vi "Licence Key Generator.vi"() -> ()   [LabVIEW 2013]
panel:
  in  "generator version":string="Version: A (proto) "
  in  "targed directory":path=path "C:/Licences"
  in  "CPU ID":string="AA13E3D1E2B87CC1" caption="Processor ID"
  in  "HDD serial":string="4J810037XGJ2AE" caption="Disk Drive Serial Number"
  in  "application name":string(combo)="Dave.exe" caption="Application name"
  in  "user name":string="Stanley Kubrick" caption="User name"
  in  "machine name":string="Hal 9000" caption="Machine name"
  in  "UUID":string="DB0CF264-5C22-497A-AB4E-F286BC2ADD07" caption="System UUID"
  in  "features":T1={"Feature 1"=TRUE, "Feature 2"=FALSE, "Feature 3"=FALSE, "Feature 4"=FALSE, "Feature 5"=FALSE, "Feature 6"=TRUE, "Feature 7"=FALSE, "Feature 8"=FALSE}
  in  "load LKRF":bool
  in  "request path":path=path "C:/LicenceRequest_B213D3E3-F046-42D3-9AC5-B825F6B790C1_Dave.txt"
  in  "cancel":bool
  in  "generate":bool
  # "Licence key target directory"
  # "Requested system informations"
  # "Feature Set (Optional)"
  # "Licence key request file"
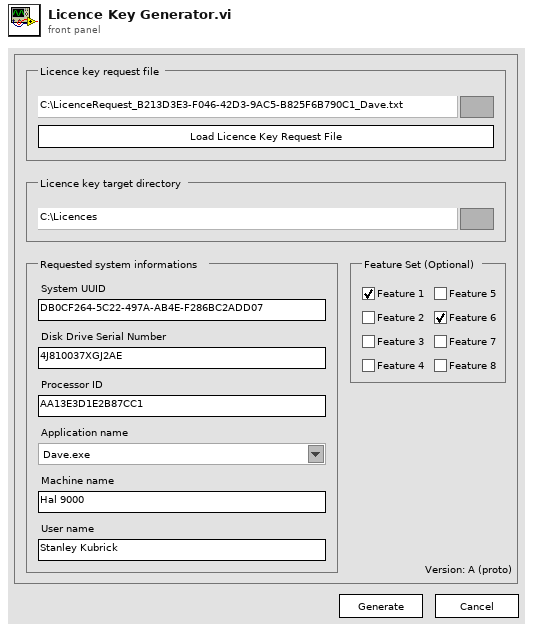
[diagram p1: front panel]
types:
  T1 = cluster{"Feature 1":bool, "Feature 2":bool, "Feature 3":bool, "Feature 4":bool, "Feature 5":bool, "Feature 6":bool, "Feature 7":bool, "Feature 8":bool}
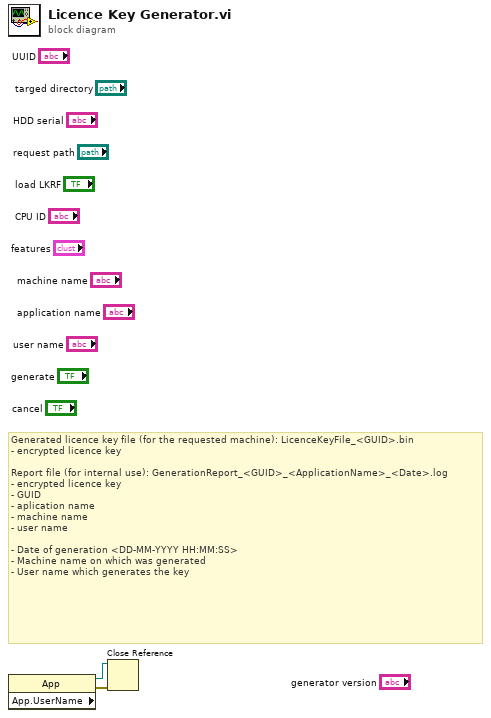
[diagram p0: block diagram]
diagram:
  # "Generated licence key file (for the requested machine): LicenceKeyFile_<GUID>.bin\n- encrypted licence key\n\nReport file (for internal use): GenerationReport_<GUID>_<ApplicationName>_<Date>.log\n- encrypted licence key\n- GUID\n- aplication name\n- machine name\n- user name\n\n- Date of generation <DD-MM-YYYY HH:MM:SS>\n- Machine name on which was generated\n- User name which generates the key"
  n1 = property class="App" props=["App.UserName"]() -> (reference out=w1:refnum<vi>, error out=w2:errorcluster)  [unwired: 2 in, 1 out]
  n2 = Close Reference(reference=w1, error in (no error)=w2) -> ()  [unwired: 1 out]
